vi "rotator.vi"(8 "Elevation":dbl, 11 "Azimuth":dbl) -> ()   [LabVIEW 2015]
uses:
  <vilib>/Utility/error.llb/DialogType.ctl
  <vilib>/Instr/_visa.llb/VISA Configure Serial Port (Instr).vi
panel:
  in  "stop":bool
  in  "Flow Control":u16(ring)=2 items=["None"=0, "XON/XOFF"=1, "RTS/CTS"=2, "DTR/DSR"=4]
  in  "Stop Bits":u16(ring)=10 items=["1.0"=10, "1.5"=15, "2.0"=20]
  in  "Parity":u16(ring) items=["None", "Odd", "Even", "Mark", "Space"]
  in  "Data bits":u16=8 min=5 max=8 step=1
  in  "VISA Resource Name":refnum<visa-resource-name>="COM3"
  in  "Baud Rate":u32=9600
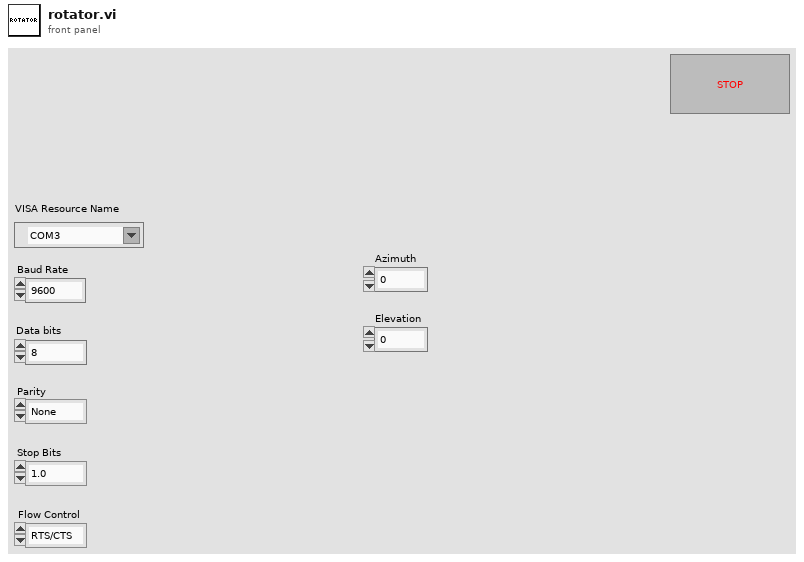
[diagram p1: front panel]
types:
  T1 = typedef "DialogType.ctl" = u16
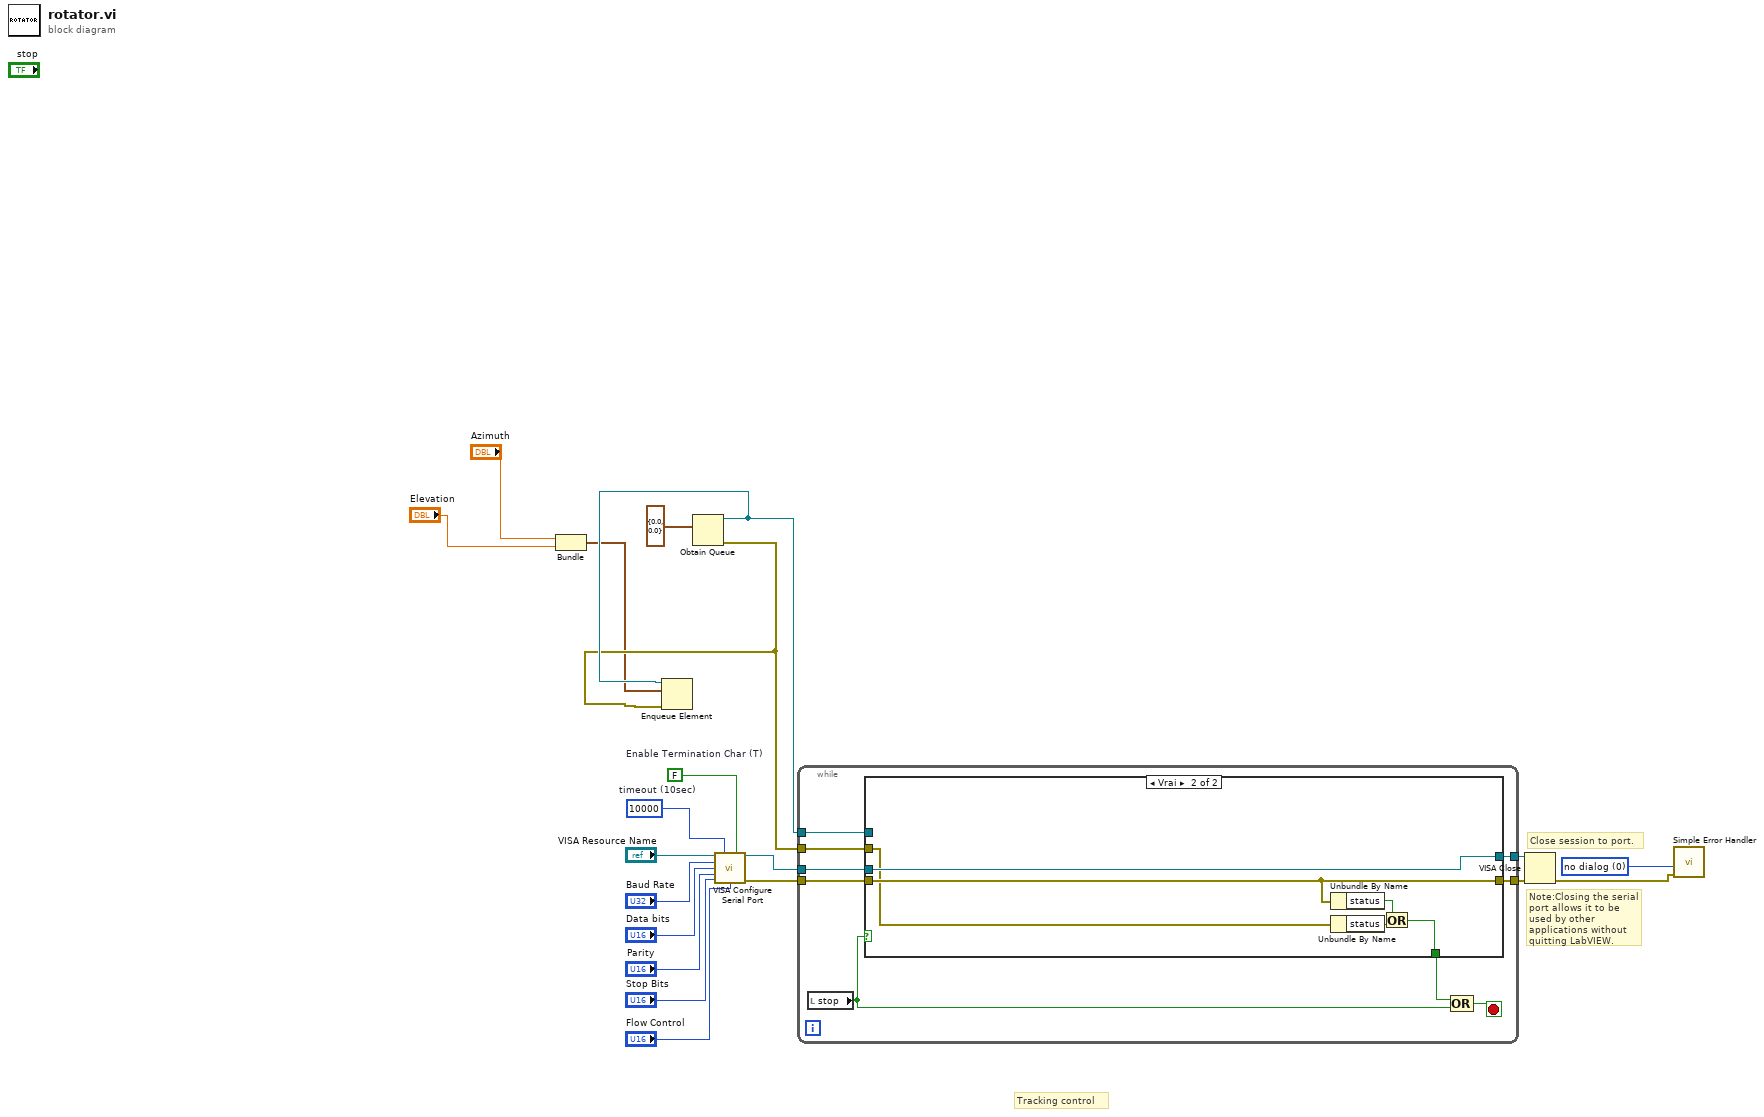
[diagram p0: block diagram]
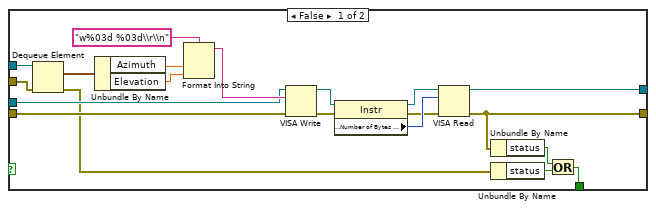
[diagram p2: hidden frame]
diagram:
  w7 = T1 0 items=["no dialog", "OK message", "continue or stop message", "OK message + warnings", "continue/stop + warnings"] ("type of dialog (OK msg:1)")
  w16 = FALSE  # Enable Termination Char (T)
  w17 = u32 10000  # timeout (10sec)
  # "Tracking control"
  # "Note:Closing the serial port allows it to be used by other applications without\nquitting LabVIEW."
  # "Close session to port."
  n1 = Bundle("Azimuth"="Azimuth", "Elevation"="Elevation") -> (w1:cluster{"Azimuth":dbl, "Elevation":dbl})  [unwired: 1 in]
  n2 = Obtain Queue(element data type=cluster{"Elevation":sgl, "Azimuth":sgl} {"Elevation"=0.0, "Azimuth"=0.0} ("output cluster")) -> (queue out=w3:refnum<queue>, error out=w2:errorcluster)  [unwired: 4 in, 1 out]
  n3 = Enqueue Element(queue=w3, element=w1, error in (no error)=w2) -> ()  [unwired: 1 in, 3 out]
  n4 = call-poly "VISA Configure Serial Port"("VISA resource name"="VISA Resource Name", "timeout (10sec)"=w17, "Enable Termination\nChar (T)"=w16, "baud rate (9600)"="Baud Rate", "data bits (8)"="Data bits", "parity (0:none)"="Parity", "stop bits (10: 1 bit)"="Stop Bits", "flow control (0:none)"="Flow Control") -> ("VISA resource name out"=w12:refnum<visa-resource-name>, "error out"=w11:errorcluster)  [unwired: 6 in]
  n5 = while {
    tunnel: w12 -> [w29]
    tunnel: w11 -> [w28]
    tunnel: [w27] -> w10
    tunnel: [w26] -> w9
    tunnel: w3 -> [w22]
    tunnel: w2 -> [w21]
    stop <- w23 stop-if-true
    n6 = local read "stop"() -> (w24:bool)
    n7 = case shown="Vrai" w24 {
      tunnel: w29 -> [w46 w55]
      tunnel: w28 -> [w45 w52]
      tunnel: [w39 w55] -> w27
      tunnel: [w33 w52] -> w26
      tunnel: [w34 w53] -> w25
      tunnel: w22 -> [w32 _]
      tunnel: w21 -> [w31 w51]
      frame False {
        n8 = Dequeue Element(queue=w32, error in (no error)=w31) -> (element=w49:cluster{"Elevation":sgl, "Azimuth":sgl}, error out=w30:errorcluster)  [unwired: 1 in, 2 out]
        n9 = Unbundle By Name(w49) -> ("Azimuth"=w35:sgl, "Elevation"=w36:sgl)
        n10 = Format Into String(format string="w%03d %03d\\r\\n", w35, w36) -> (resulting string=w47:string)  [unwired: 2 in, 1 out]
        n11 = VISA Write(VISA resource name=w46, write buffer=w47, error in (no error)=w45) -> (VISA resource name out=w41:refnum<visa-resource-name>, error out=w40:errorcluster)  [unwired: 1 out]
        n12 = property class="Instr"(reference=w41, error in=w40) -> (reference out=w42:refnum<visa-resource-name>, error out=w43:errorcluster, "Serial Settings:Number of Bytes at Serial Port"=w44:u32)
        n13 = VISA Read(VISA resource name=w42, byte count=w44, error in (no error)=w43) -> (VISA resource name out=w39:refnum<visa-resource-name>, error out=w33:errorcluster)  [unwired: 2 out]
        n14 = Unbundle By Name(w33) -> ("status"=w38:bool)
        n15 = Unbundle By Name(w30) -> ("status"=w37:bool)
        n16 = Or(x=w38, y=w37) -> (x .or. y?=w34:bool)
      }
      frame True {
        n17 = Unbundle By Name(w52) -> ("status"=w54:bool)
        n18 = Unbundle By Name(w51) -> ("status"=w50:bool)
        n19 = Or(x=w54, y=w50) -> (x .or. y?=w53:bool)
      }
    }
    n20 = Compound Arithmetic op=OR(w25, w24) -> (w23:bool)
  }
  n21 = VISA Close(VISA resource name=w10, error in (no error)=w9) -> (error out=w8:errorcluster)
  n22 = call <vilib>:"Simple Error Handler.vi"("type of dialog (OK msg:1)"=w7, "error in (no error)"=w8) -> ()  [unwired: 3 in, 5 out]
